vi "MergeData.vi"() -> ()   [LabVIEW 2022 SP3]
uses:
  <vilib>/Utility/file.llb/Read From Spreadsheet File (DBL).vi
  <vilib>/Utility/file.llb/Write To Spreadsheet File (DBL).vi
panel:
  out "Bwidth Data":sgl[][](array[numeric])
  in  "Bandwidth Data":bool
  in  "Merge Data":bool
  out "center freq":sgl format="%.2f"
  out "XY Graph":cluster{"all rows":dbl[], "all rows":dbl[]}(graph)
  in  "Save spectrum only":bool
  out "bandwidth":sgl format="%.2f"
  out "upper band freq":sgl format="%.2f"
  out "lower band freq":sgl format="%.2f"
  in  "dB width pt":dbl=-15.0 format="%.2f"
  out "max f":sgl format="%.2f"
  out "max freq (dB)":sgl format="%.2f"
  out "transposed array":sgl[][](array[numeric])
  in  "pattern":string
  in  "Use Selected Files":bool
  in  "Listbox":i32[](listbox)
  in  "Choose Directory":path
  # "© 2000 Riverside Research Institute"
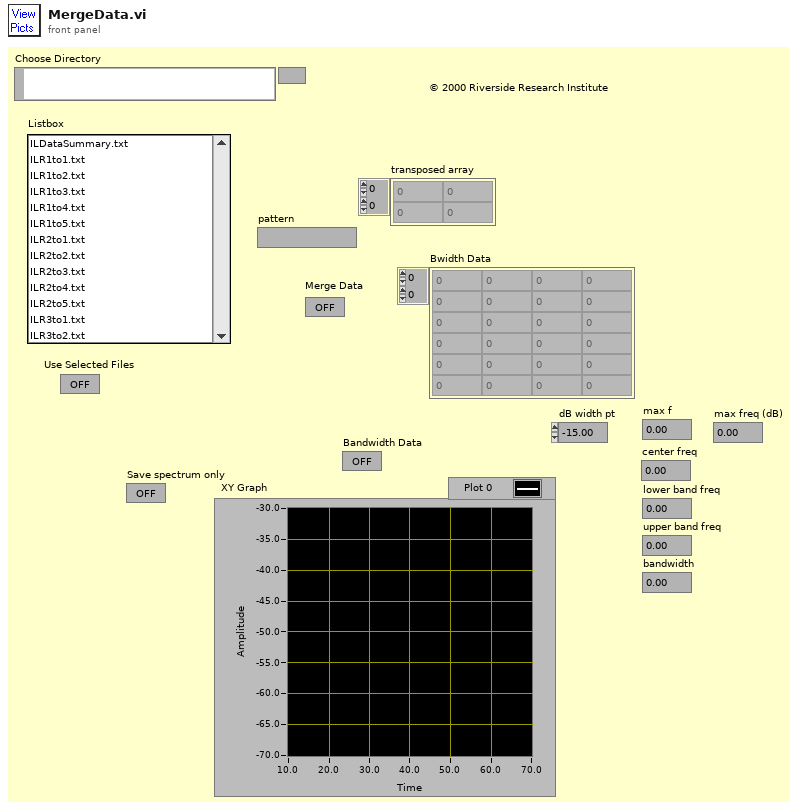
[diagram p1: front panel]
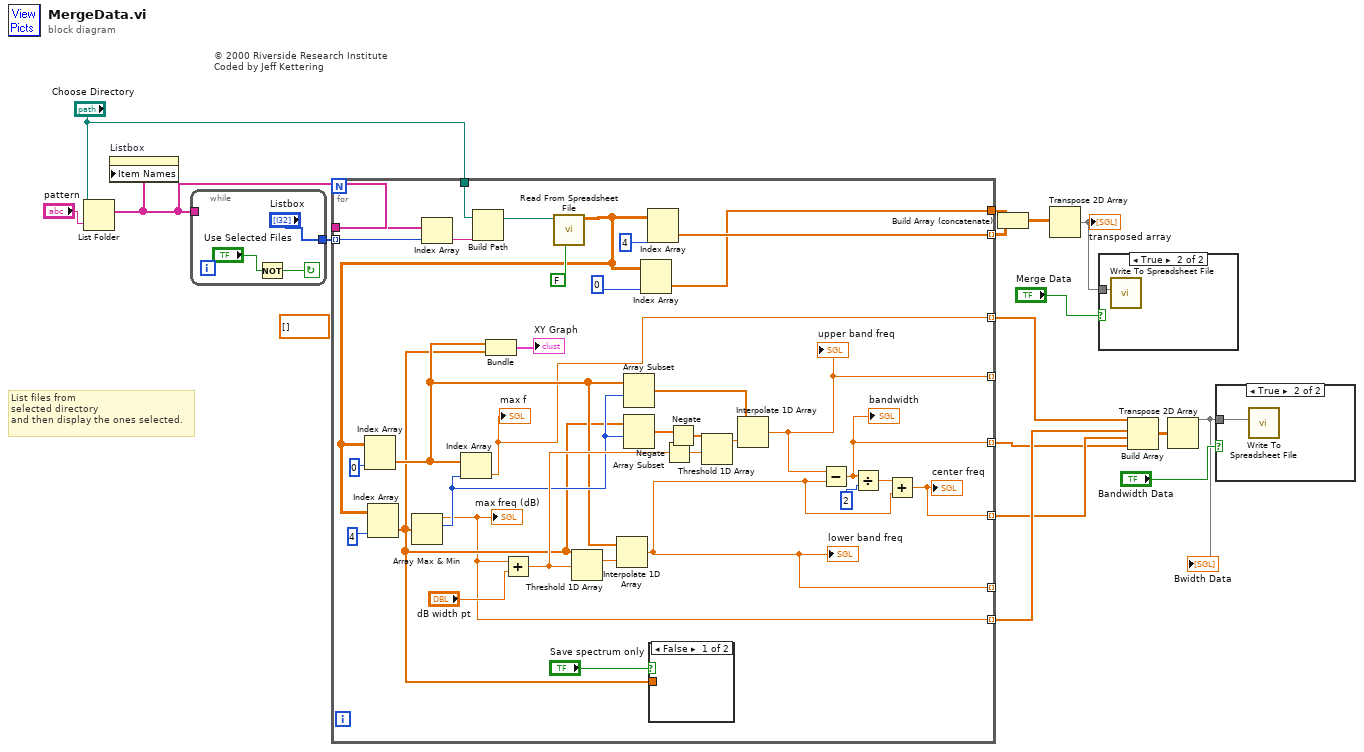
[diagram p0: block diagram]
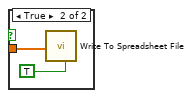
[diagram p4: hidden frame]
diagram:
  (unwired) dbl[] [] ("transposed array")
  # "© 2000 Riverside Research Institute\nCoded by Jeff Kettering"
  # "List files from\nselected directory\nand then display the ones selected."
  n1 = List Folder(path="Choose Directory", pattern="pattern") -> (filenames=w15:string[])  [unwired: 1 in, 4 out]
  n2 = property on="Listbox" class="LstBox (strict)"("Item Names"=w15) -> ()  [unwired: 2 in, 2 out]
  n3 = while {
    tunnel: w15 -> [_]
    tunnel: ["Listbox"] -> w16
    stop <- w18 continue-if-true
    n4 = Not(x="Use Selected Files") -> (.not. x?=w18:bool)
  }
  n5 = for {
    tunnel: "Choose Directory" -> [w51]
    tunnel: w16 -> [w53] mode=indexing
    tunnel: w15 -> [w52]
    tunnel: [w47] -> w11 mode=indexing
    tunnel: [w44] -> w12
    tunnel: [w25] -> _ mode=indexing
    tunnel: [w24] -> w5 mode=indexing
    tunnel: [w23] -> w6 mode=indexing
    tunnel: [w22] -> w8 mode=indexing
    tunnel: [w21] -> _ mode=indexing
    tunnel: [w20] -> w7 mode=indexing
    n6 = Index Array(array=w52, index=w53) -> (element=w50:string)
    n7 = Build Path(base path=w51, name or relative path=w50) -> (appended path=w49:path)
    n8 = call-poly <vilib>:"Read From Spreadsheet File.vi"("transpose (no:F)"=FALSE, "file path (dialog if empty)"=w49) -> ("all rows"=w26:dbl[][])  [unwired: 2 in, 7 out]
    n9 = Index Array(array=w26, index (col)=0) -> (element=w31:dbl[])  [unwired: 1 in]
    n10 = Index Array(array=w26, index (col)=4) -> (element=w30:dbl[])  [unwired: 1 in]
    n11 = Array Max & Min(array=w30) -> (max value=w20:dbl, max index (indices)=w35:i32)  [unwired: 2 out]
    "max freq (dB)" <- w20
    n12 = Index Array(array=w31, index=w35) -> (element=w22:dbl)
    "max f" <- w22
    n13 = Bundle("all rows"=w31, "all rows"=w30) -> (→"XY Graph":cluster{"all rows":dbl[], "all rows":dbl[]})  [unwired: 1 out]
    n14 = Add(x=w20, y="dB width pt") -> (x+y=w38:dbl)
    n15 = Threshold 1D Array(2:w38, 3:w30) -> (0:w40:dbl)  [unwired: 1 out]
    n16 = Interpolate 1D Array(1:w40, 2:w31) -> (0:w21:dbl)
    "lower band freq" <- w21
    n17 = Array Subset(array=w31, index=w35) -> (w36:dbl[])  [unwired: 1 in]
    n18 = Array Subset(array=w30, index=w35) -> (w33:dbl[])  [unwired: 1 in]
    n19 = Index Array(array=w26, index (col)=0) -> (element=w44:dbl[])  [unwired: 1 in]
    n20 = Index Array(array=w26, index (col)=4) -> (element=w47:dbl[])  [unwired: 1 in]
    n21 = case shown="False" "Save spectrum only" {
      tunnel: w30 -> [_ w55]
      frame False {
      }
      frame True {
        n22 = call-poly <vilib>:"Write To Spreadsheet File.vi"("transpose? (no:F)"=TRUE, "1D data"=w55) -> ()  [unwired: 4 in, 3 out]
      }
    }
    n23 = Negate(x=w38) -> (-x=w32:dbl)
    n24 = Negate(x=w33) -> (-x=w34:dbl[])
    n25 = Threshold 1D Array(2:w32, 3:w34) -> (0:w39:dbl)  [unwired: 1 out]
    n26 = Interpolate 1D Array(1:w39, 2:w36) -> (0:w25:dbl)
    "upper band freq" <- w25
    n27 = Subtract(x=w25, y=w21) -> (x-y=w24:dbl)
    "bandwidth" <- w24
    n28 = Divide(x=w24, y=2) -> (x/y=w27:dbl)
    n29 = Add(x=w27, y=w21) -> (x+y=w23:dbl)
    "center freq" <- w23
  }
  n30 = Build Array (concatenate)(w12, w11) -> (w10:dbl[][])
  n31 = Transpose 2D Array(2D array=w10) -> (transposed array=w9:dbl[][])
  "transposed array" <- w9
  n32 = case shown="True" "Merge Data" {
    tunnel: w9 -> [_ w56]
    frame False {
    }
    frame True {
      n33 = call-poly <vilib>:"Write To Spreadsheet File.vi"("2D data"=w56) -> ()  [unwired: 5 in, 3 out]
    }
  }
  n34 = Build Array(w8, w7, w6, w5) -> (w3:dbl[][])
  n35 = Transpose 2D Array(2D array=w3) -> (transposed array=w1:dbl[][])
  "Bwidth Data" <- w1
  n36 = case shown="True" "Bandwidth Data" {
    tunnel: w1 -> [_ w57]
    frame False {
    }
    frame True {
      n37 = call-poly <vilib>:"Write To Spreadsheet File.vi"("2D data"=w57) -> ()  [unwired: 5 in, 3 out]
    }
  }
